vi "SolarArrayCalculator.vi"() -> ()   [LabVIEW 2015]
panel:
  out "Waveform Graph":dbl[](graph)
  in  "String 5":string
  in  "String 4":string
  in  "String 3":string
  in  "String 2":string
  in  "String":string
  out "E   in Wattt per nyear":dbl
  in  "PR":dbl
  in  "H":dbl format="%#_13g"
  in  "r":dbl
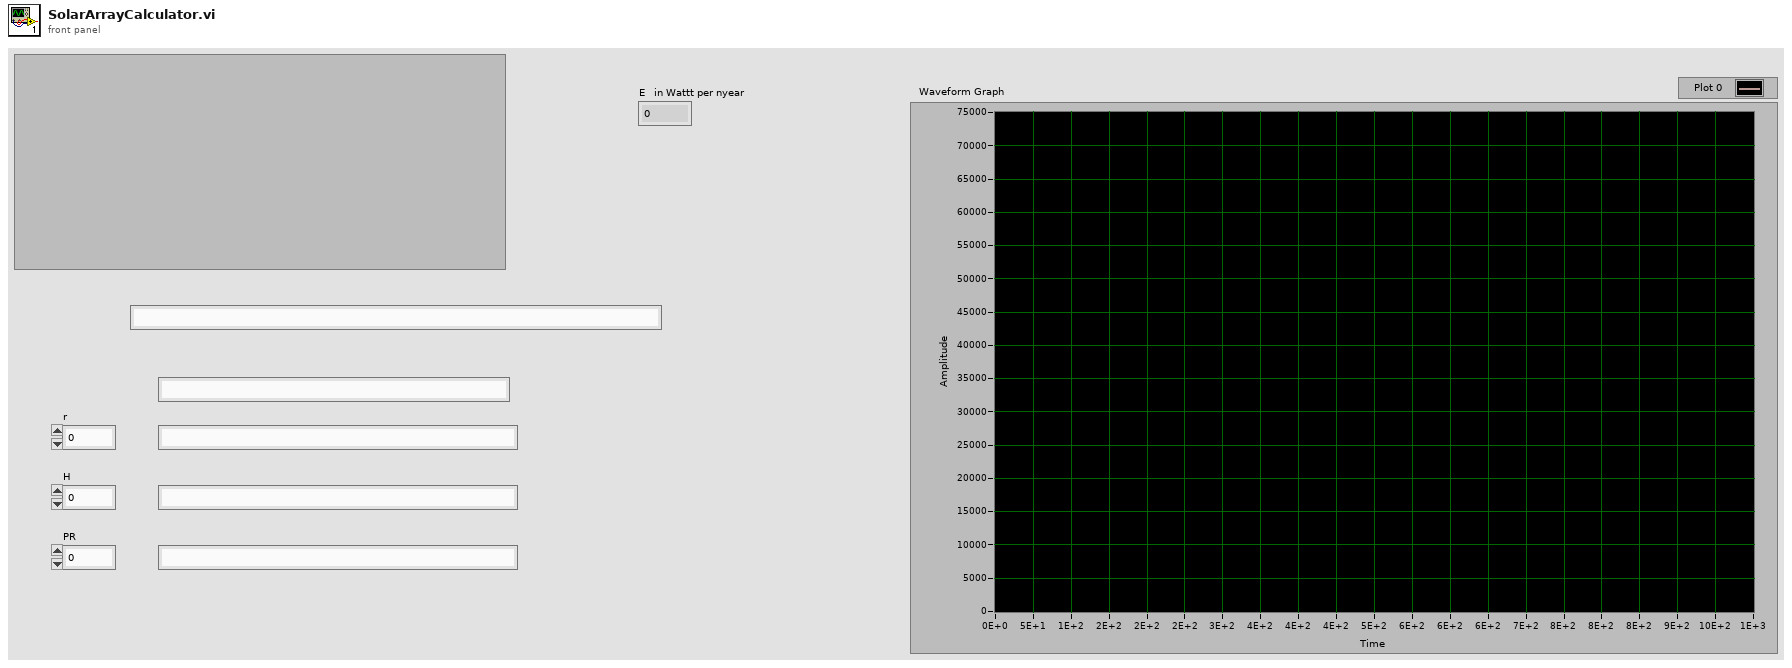
[diagram p1: front panel]
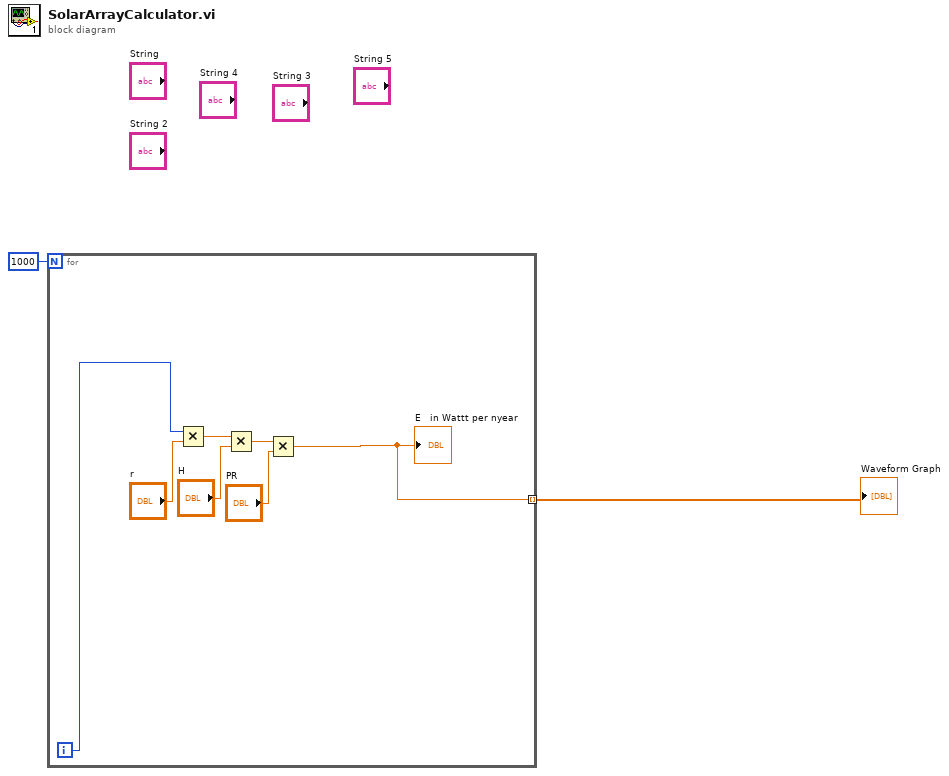
[diagram p0: block diagram]
diagram:
  n1 = for {
    N: 1000 -> [_]
    tunnel: [w3] -> w1 mode=indexing
    i -> [w4]
    n2 = Multiply(x=w4, y="r") -> (x*y=w9:dbl)
    n3 = Multiply(x=w9, y="H") -> (x*y=w6:dbl)
    n4 = Multiply(x=w6, y="PR") -> (x*y=w3:dbl)
    "E   in Wattt per nyear" <- w3
  }
  "Waveform Graph" <- w1
